vi "Sample Push Reset to Idle.vi"(6 "Echo (True)":bool=TRUE, 8 "error in (no error)":errorcluster, 11 "cRIO-CO2 in":refnum<class "cRIO-CO2.lvclass">) -> (0 "error out":errorcluster, 3 "cRIO-CO2 out":refnum<class "cRIO-CO2.lvclass">)   [LabVIEW 2015, in "cRIO-Carbondioxide.lvlib" / "cRIO-CO2.lvlib" / "cRIO-CO2.lvclass"]
uses:
  cRIO-CO2.lvclass
  Controls/Sample Push State Enumerator.ctl
  subs/Sample/Sample.lvclass
  <vilib>/ActorFramework/Time-Delayed Send Message/Time-Delay Override Options.ctl
  cRIO-CO2.lvclass/cRIO-CO2.ctl
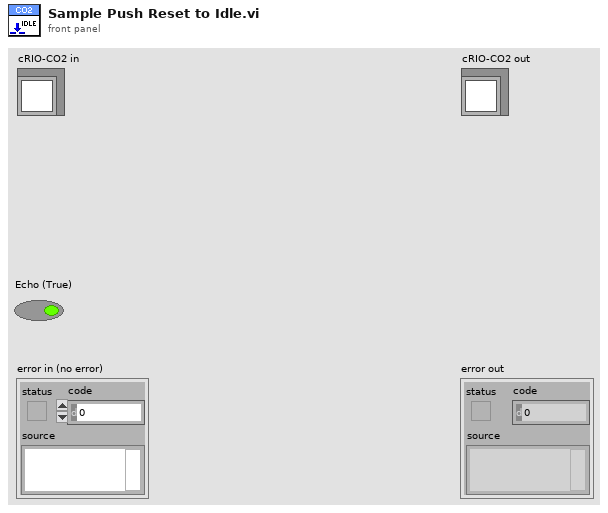
[diagram p1: front panel]
types:
  T1 = typedef "Time-Delay Override Options.ctl" = enum16{"Send next copy now", "Skip next scheduled copy", "Send next copy now and stop all further copies", "Stop all further copies"}
  T2 = typedef "Sample Push State Enumerator.ctl" = enum16{"Undefined", "Initialize", "Dilute", "Close Transfer Line", "Start Heaters", "Warm Up Syringe", "Ready to Push", "Push", "Initiate Stash", "Stash", "Complete", "Abort", "Idle", "Error"}
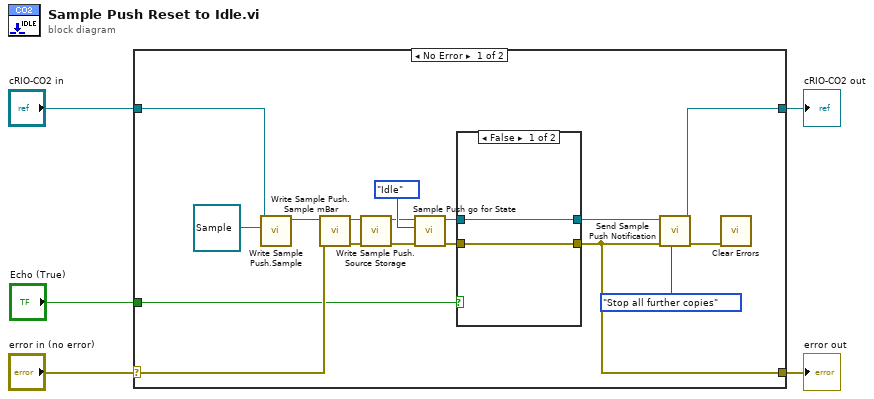
[diagram p0: block diagram]
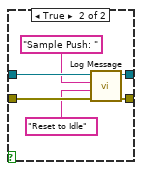
[diagram p2: hidden frame]
diagram:
  n1 = case shown="No Error" "error in (no error)" {
    selector: "error in (no error)" -> [w9 w32]
    tunnel: [w7 w32] -> w4
    tunnel: [w20 w31] -> w2
    tunnel: "cRIO-CO2 in" -> [w8 w31]
    tunnel: "Echo (True)" -> [w6 _]
    frame No Error {
      n2 = call "Write Sample Push.Sample.vi"("Sample.lvclass"=refnum<class "Sample.lvclass"> refnum ("Sample Push.Sample"), "cRIO-CO2 in"=w8) -> ("cRIO-CO2 out"=w11:refnum<class "cRIO-CO2.lvclass">)  [unwired: 9 in]
      n3 = call "Write Sample Push.Sample mBar.vi"("error in (no error)"=w9, "cRIO-CO2 in"=w11) -> ("error out"=w10:errorcluster, "cRIO-CO2 out"=w13:refnum<class "cRIO-CO2.lvclass">)  [unwired: 8 in]
      n4 = call "Write Sample Push.Source Storage.vi"("error in (no error)"=w10, "cRIO-CO2 in"=w13) -> ("error out"=w14:errorcluster, "cRIO-CO2 out"=w12:refnum<class "cRIO-CO2.lvclass">)  [unwired: 8 in]
      n5 = call "Sample Push go for State.vi"("error in (no error)"=w14, "Sample Push State"=Sample_Push_State_Enumerator."Idle", "cRIO-CO2 in"=w12) -> ("error out"=w18:errorcluster, "cRIO-CO2 out"=w17:refnum<class "cRIO-CO2.lvclass">)  [unwired: 7 in]
      n6 = case shown="False" w6 {
        tunnel: w18 -> [w23 w30]
        tunnel: w17 -> [w24 w29]
        tunnel: [w24 w26] -> w16
        tunnel: [w23 w25] -> w7
        frame False {
        }
        frame True {
          n7 = call "Log Message.vi"("error in (no error)"=w30, "String"="Reset to Idle", "Source Name"="Sample Push: ", "cRIO-CO2 in"=w29) -> ("error out"=w25:errorcluster, "cRIO-CO2 out"=w26:refnum<class "cRIO-CO2.lvclass">)  [unwired: 6 in]
        }
      }
      n8 = call "Send Sample Push Notification.vi"("notification (Send next copy now)"=Time-Delay_Override_Options."Stop all further copies", "error in (no error)"=w7, "cRIO-CO2 in"=w16) -> ("error out"=w22:errorcluster, "cRIO-CO2 out"=w20:refnum<class "cRIO-CO2.lvclass">)  [unwired: 7 in]
      n9 = call <vilib>:"Clear Errors.vi"("error in (no error)"=w22) -> ()  [unwired: 5 in, 2 out]
    }
    frame Error {
    }
  }
  "error out" <- w4
  "cRIO-CO2 out" <- w2
